vi "Day 10 Task 1 and 2.vi"() -> ()   [LabVIEW 2018]
panel:
  out "Middle score pt2":u64
  out "Scores of incomplete":u64[](array[numeric])
  out "Size of input":i32
  out "Total score pt 1":i64
  out "Scores":i32[](array[numeric])
  out "Error reason":string[](array[string])
  out "Error":bool[](array[boolean])
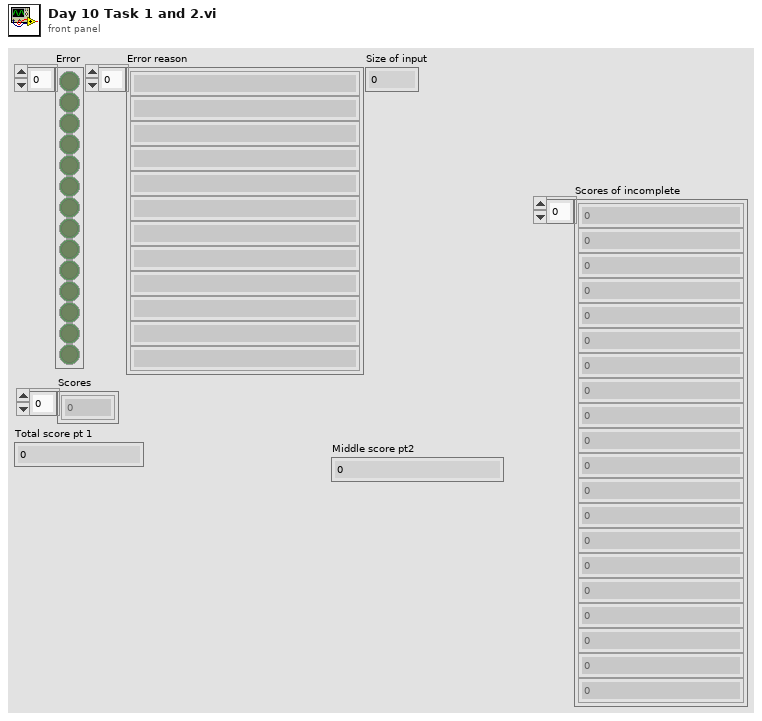
[diagram p1: front panel]
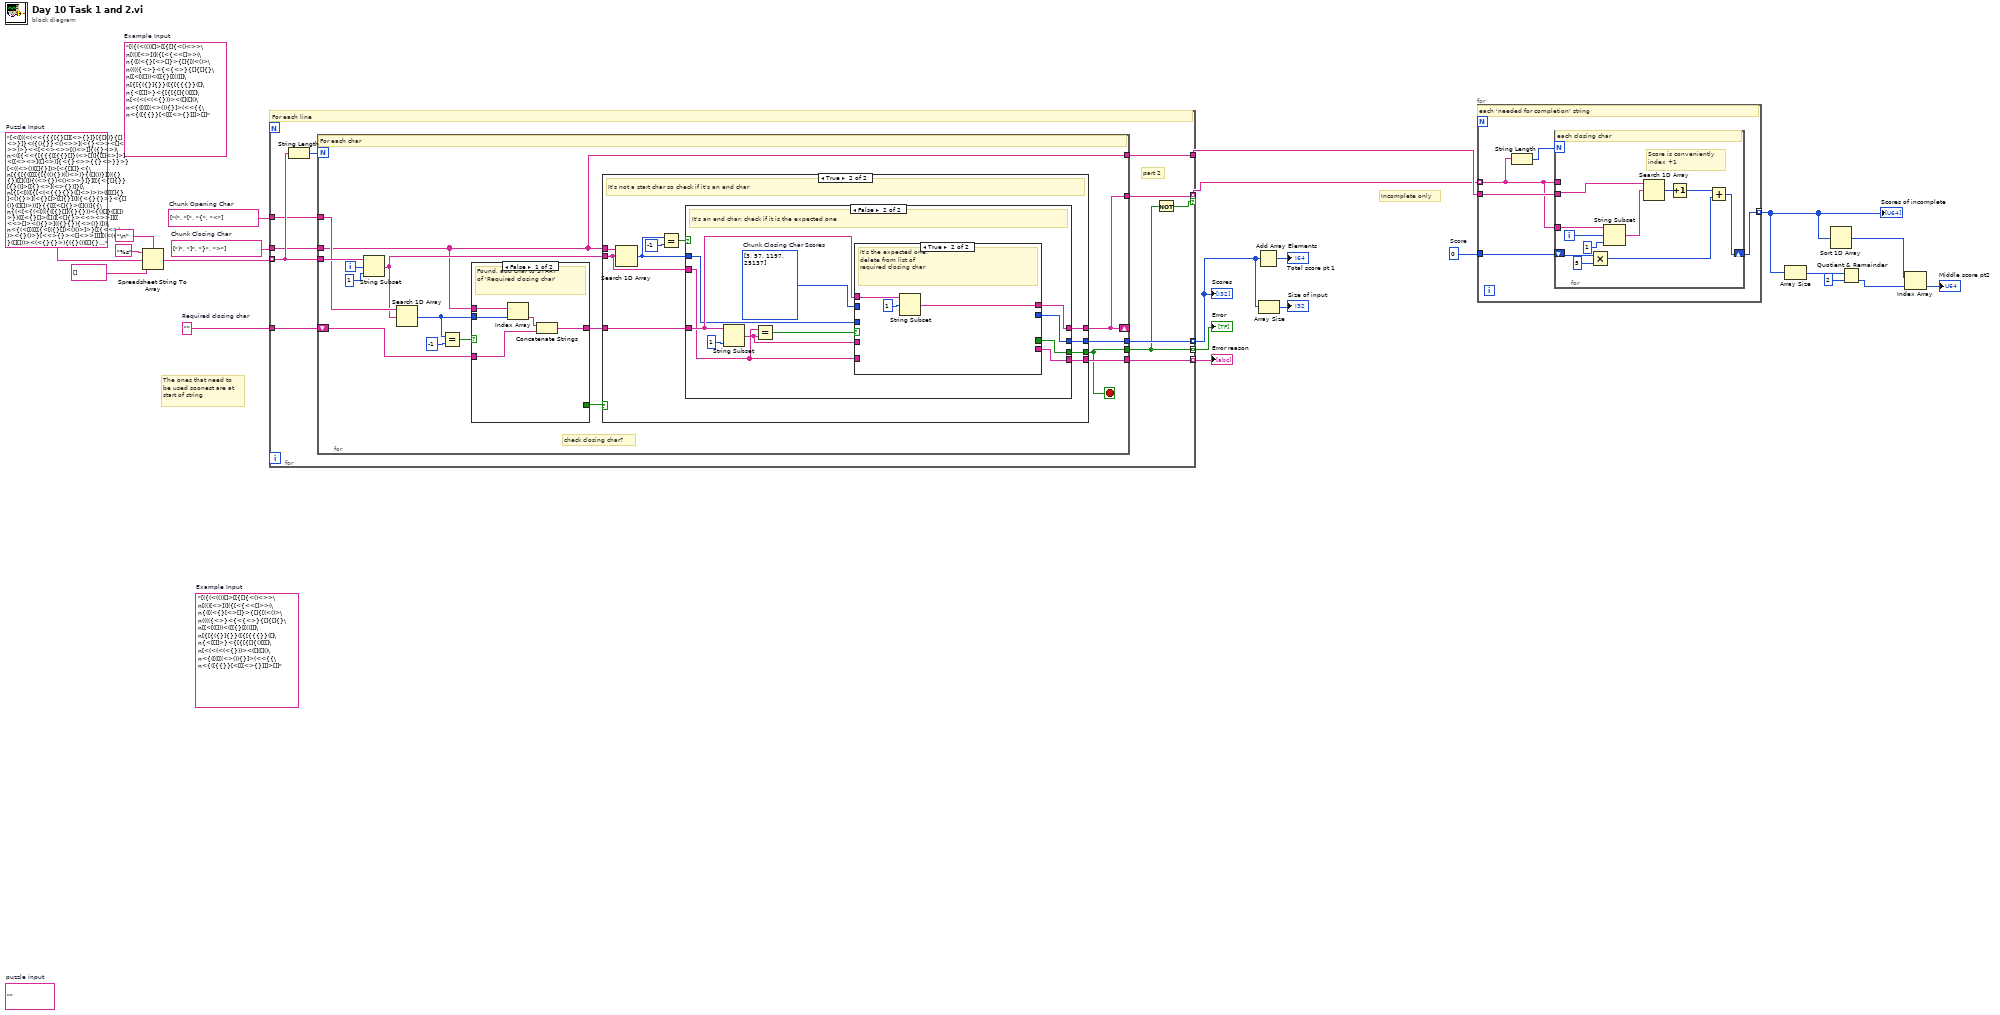
[diagram p0: block diagram]
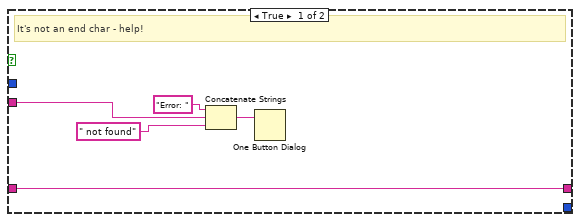
[diagram p3: hidden frame]
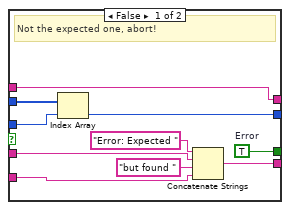
[diagram p4: hidden frame]
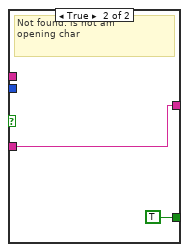
[diagram p5: hidden frame]
diagram:
  w8 = u64 0  # Score
  (unwired) "[({(<(())[]>[[{[]{<()<>>\n[(()[<>])]({[<{<<[]>>(\n{([(<{}[<>[]}>{[]{[(<()>\n(((({<>}<{<{<>}{[]{[]{}\n[[<[([]))<([[{}[[()]]]\n[{[{({}]{}}([{[{{{}}([]\n{<[[]]>}<{[{[{[]{()[[[]\n[<(<(<(<{}))><([]([]()\n<{([([[(<>()){}]>(<<{{\n<{([{{}}[<[[[<>{}]]]>[]]"  # Example Input
  w12 = ""  # Required closing char
  w1 = "[<([((<(<<{{{[{}[]][<>{}]}[{[]()}{[]<>}]}<({(){}}<()<>>](<{}<>><[]<>>)>}<<[<<><>>[()<>]]{({}<>)\n<([{<<{[{{{[[{{}[]}(<>[])]{[[]<>]>]<[[<><>]([]<>)]{<{}<>>{{}<>}}>}[<((<>())[[]{}])>[<{[][]}<{\n[{{[{([[[[{[{((){})(()<>)}{([]())}][(({}{})[[]()]){(<>{})<()<>>}]}][[{<{[]{}}[{}()]>[[{}<>](<>{})]}[\n[{[<[(([{[<(<{{}{}}([]<>)>)>([[[[]{}]<(){}>](<{}[]>[[]{}])]({<{}{}>}<{[]()}([][])>))]}{{[[[<[]{}>([]())]{{\n{(<[<{(<[(({([{}[]]({}{}))<{()[]}([][])>})([[<{}[]>([])][<[]{}><<><>>]][[<<>[]><(){}>](({}{}){<>()})]))\n<{(<[[([[[{<[({}[])<()()>]>}[[{<<>()><{}()>}[<<>{}><[]<>>]]]][(<({[]}([][]))><(<{}{}>){({}())[[]{}]}>){[[\n(<(<(((<<{[<[{[]{}}({}{}>]><[<()<>><{}{}>][{()<>}({}())]>]}({<[[[]()]{[]<>}](<[]<>>([]<>))>[{(<><>)([][])}]\n<{[[{({<([[<{(<>())[<>[]]}><({[]{}}<<>>)[((){})[[]()]]>]]({<<(<><>)[{}<>]>{[{}{}](()[])}>([([]<>){()\n(((<{{{{<<[<([[]<>])({()<>}[{}<>])>(<{<>()}>{[{}<>]})]><[[([[]{}]{{}()})(([]){(){}})]{[{<>{}}<<>{}>\n[{((({[[([[[{{[]<>}(<>[])}[([]{})([][])}]<[(<><>){[][]}]{<{}{}>(()())}>]]<([<{{}()}{{}<>}>[(\n{(<{[[{(<[[{{[(){}](()[])}}<[(<>{}){[][]}]{<<><>>{{}()}}>][{{{()}<()()>}{<<>()>(()[])}}]]>[{<({[<>\n(([([([(([<([([][])<()()>]<({}()]({}())>)>{[{<[][]>(<>{})}<{{}{}}(<>{})>]<{([]())(<>{})}[{<>{}}[()()]]\n{<<<{[({(<({(<{}()>){[<>()](()<>)}})<[<{()[]}{<><>}>]{[[(){}]({}<>)][<<>{}><{}<>>]}>><(([<{}[]>(<>\n{[[([[([{[(<<(<>[]){{}}><([]<>)<()<>>>><([(){}](<>{}))[{[]}<{}<>>]>)][{{(({}())[[]{}])}{([()<>][[]<>]){<[][]>\n{([{(({<<{<{{(<>())[{}{}]}{(()[])[[]<>]}}>}>[<{(<[[]()]<{}()>>)<{((){}]((){})}[[{}]([]{})]>}([({\n(([(<({[<({{<{<>[]}<<>{}>](([]()))}<(<{}()>(<>))<((){})[<>{}]>>})({[[<()<>>][<()<>>[<><>]]](({\n<<((<<{[{(<<<{{}{}}[{}<>])(<<>()>[[][]])>>([({()[]}[<>{}]){[{}<>]{()<>}}]{(<{}{}>[<>[]])[{<>[]}<[]{\n([{(<<{{<{<<<<()<>>([][])>(([]()){()})><{[{}()]{<>{}}}<{()<>}<()[]]>>>}{<<<{()}((){})>[[{}()][<>]]>>[\n<[(<<<([{{{((<()>(<>{}))<([]<>)(<>())>){([(){}]<()()>)}}{{[[()[]](()<>)]{(<>()){()()}}}<[({}()){[]<>}][<{}[\n(<{{({({({[{([()<>])[{<>{}}]}{<([]())[[]<>]>([()()]{[]<>})}]{(<[{}()]<<>()>>[<<>())<()[]>])[({()()}[[]\n<({<({[{(({{{<{}()>[(){}]}{({}<>)<[]{}>}}<<<{}[]>([]<>)>[(()())[()<>]]>}<(<[[]{}]([]())>([(){}]<[][]\n{(((<(<{{{<[[{[][]}]<{[]{})[{}()]>]<[<{}<>>][[[]()](()<>)]>>}([([{{}[]}[<>[]]][(<>{}){[]()}])({[{}[]][<>\n{{({(<{{(([<(<()<>>{(){}})>[<{()()}[<>{}]>[<<>{}>{[][]}]]]({{<<><>><[][]>}[[<>()]<[]()>>}<<(()())[[]<>]><{<\n<{(<([{[{<[[[(<>)({}{})]]((<()<>>))]{{{(()<>)([])}}[{{{}()}{<>[]}}[{[]{}}{<><>}]]}>}][<[<[<[(){}]><({}[])<<>{\n<({[[<<([(<{[<[]<>>[{}<>]](({}[]))}{{[{}<>]}([[]{}]([]{}))}>[[{<[]<>)<{}>}{{(){}}{()}}]([(<>{})]<<[]()>\n{(([{<{(((<<<(()[])([]())>[<<>{}>({}[]]]>>[[([[]<>]<{}[]>)<[<>[]]{(){}}>][((<>[])(()[]))]]))(([{<{<>}{{}<>\n<[((([<{{([{({<>{}}(<><>)){([]{})<()[]>}}({[[][]]([]{})}({[]<>}))][<<[<>{}]([][])>(<{}<>>[(\n<[{{[{{<{[[([<<><>>]{({}())([]<>)})]]}[<({([{}{}]{[]})({()()}[(){}])}[{<(){}><{}[]>}])<[[<[]{}>\n(<(<{<{<{([([<<><>>]({[]}[()[]])){<{<>()}<()[]>>[([]{}){{}[]}]}]{{({[]()}{<><>})([{}()](()()))}<[<[][]>][<[]\n{[{{<[(<(<{<{{<><>}{{}{}}}([()()])>[<<{}>[()()]>[[()()]{[][]}]]}>)[<<<<<[]()><(){}>>[[<>()]<{}{}>]>[{{\n([{(<({((([<(<()()><[]()>)({{}()}{<>()})>{[({}[]){{}[]}]{{{}()}{{}<>}}}])(<[{((){}){[][]}}([[]()])]{<{()<>\n((<<[{<[(([({(()<>)[{}{}]}{<{}[]><[]<>>})<[<()>]([()<>])>]{((<[]{}><()<>>)<{{}><<>>>)[(<{}()>)<[[]()](\n({<([[<{[{[[{{{}<>}({}())}<[<>()][{}[]]]][[{[]<>}]<([]{})[{}()]>]]}]([{[(<[]{}>[{}[]])]}]{((<[{}\n<[(<{<[<<({<<{<><>}(()())>)}{(({(){}}){[{}[]]{{}{}}})})>>]>}<[<{(<<[(<()<>>[[]()]){{{}<>}<[][]>}][(<(\n({([(<{[{[{<({<>{}}<()[]>)>{[(<><>){{}<>}]}}]}]}[([[{[[[[]{}]][([][]){<>{}}]][[{[][]}(<>[])]\n[<([<[([[{{({{<>{}}[{}[]]}([()()]({})))((<(){}>)([[]())({}<>)))}}]])]>{<<(({{<[<{}[]>[()<>]]>}}([[{({}<>)\n<{[{<[<([{(<{<<>{}><<>()>}[(<>[])[<><>]]>[(((){}))<(<>){{}[]}>]){(<({}{})[{}{}]}<<[]{}><{}<>>>\n{[[{<{[<<<(<<(<><>)<[][]>>{[<>{}]{()<>}}>{{{[]<>}<<>()>}}){(<{<>()}(()<>)>{{{}[]}(()())})]>>({(([<{}()>([]{\n[<({(({<<{<<{<<>>{<><>}}((<>{})({}()))>([({}())([][])][{{}{}}<[]<>>])>}((<<<(){}>{{}()}>[{<>()}({}{\n<([[[{[(({([{<()<>>}]{(([]<>)[()<>])}){<[{()()}[<><>]]([<><>][{}[]])>{({{}{}}){<{}[]><<><>>}}}}{<({<()<>\n<[<((<[[<({{[{<><>}{{}{}}]{<{}{}><(){}>}}{{[[]{}][<>[]]}([<><>][{}()])}}({{{<>()}<<>{}>}([{}]{\n{[(<({[{<<{<{{()[]}({}())}{{{}()}<()>}>[<([]{})<<>{}>><{{}()}{{}{}}>]}<{({[][]}{{}[]})}<<{<>{}}[[][]]>>>>\n<{[<([(<<([[(<[]<>><{}()>)<({}<>){(){}}>]]<<[(<>{}){{}<>}]([[]{}]({}{}))>>)>{[{[<<[]><{}<>>>(({}{}))\n{(<<{{{((<<[({[][]})[([]())(<>{})]][((()<>)([][]))}><([[()[]]]){<<[][]>><<{}[]>[(){}]>}>>[([{[[]<\n<{(<<<{{((<{{<{}()>[<>()]}({<>{}}[(){}])}[{({}<>)(()[])}<{(){}}<{}{}>>]>{{[[[]{}]<[][]>]{[{}{}][[]<>]}\n{(<(<([{<([<{{<>}<<>{}>}{<()[]>[[]()]}>{<[()()]({}{})>((<>{}))}][{<{[]}[[]()]>{{<>}[[]<>]}}({<<>{}>[[][]]}{<\n{((<[<<[{<{[{{{}<>}}<[<>()]([]())>]([<()()><()()>]{[()<>]{[]()}})}<{([[]()]{<>})}(<<[]{}}{[][\n[{{{<<<[{[(<[{[]{}}{(){}}}(<()>[[][]])>{{(<><>)<<>()>}<<<>{}>(())>})]{<(<<[]()>({}())><[{}<>]{[]()}>)><\n{{[[[({((({{({{}()}<()()>)}{(<{}{}>{()<>})[(()<>)<<><>>]}}<[<[{}[]][()<>]>[[(){}][()()]]>{<{<>[]}[\n[<[([{[{[{[{({(){}})}[[<[]{}>{<>()}]]]<[<{<>()}[<><>]>[{<>[]}<()()>]][<{[]{}}({}())>{<[]()>{{}()}}]>\n<([{({<(({<{<[[]{}]({}[])>[[<>[]]<<>[]>]}>}{(({(()[])[[]()]})<[[{}<>][<>{}]]<[[]()]([])>>)}))[([[([([][])[<\n{<{[([(({<(<{{<>[]}[[]<>]}<(<><>)[[]{}]>>{{{{}()}((){})}))<[{[{}{}]([]{})}{([]())(<>{})}][<(()[])\n([[[([<[[{{((<{}{}>(<>()))[({}[]){<>{}}])}}[[(({{}{}}(()[]))<[<>{}]<()<>>>)]<({<()<>>}{{{}<>}{(\n(<([{[{<[{[<<<{}()}{{}<>}>({(){}}<[][]>)><{<<>[]>((){})}>](<([()()])[([])({}{})]>[[<{}[]>(<>\n([(<{<([{{[[[({}{})[(){}]]]([(()<>)[<>[]]][<{}{}>])][<[<<>[]>[(){}]][[{}[]](<>[])]>({{{}[]>([]{})}[{[][]}[{}\n{<[(<[({[<({[({}[])]<{{}<>}[{}()]>}<{{{}{}}[[]]}<(()())[[]<>]>>)>{[{[(<>{})[<>{}]]<({}<>)((){})\n{[{[<<<[([[[<{[]{}}[<>()]>(([][])({}[]))]<[[<>()]{<>()}]<[()[]]{[]()}>>]](<{<[()[]]>{({}{})}}(<<[]<>><[]<>>\n({[<{{<<({<(<[{}{}]>)[(<{}{}>[[]{}]){<{}()>{<>[]}}]>(({<<><>><<><>>}({[][]}))[[{{}}([]{})]])}[({(<{}[]>{()<>}\n({{{{{{[<[<([([]){{}[]}][([]{})])(<([]{})(<>{})><[<>](()())>)>{(([[]()](()())))}]{[[({()[]}{<>(\n(({{[<[[[((<{(()<>)[[]{}]}([[]()]{<><>})>))((<{{(){}}(<>())}(<<><>><[]{}>)>(({()()}[{}[]])))<([<<>><()[]>])<\n<[[{<({[((<<({{}()}{<><>})<<()[]>[{}()]>>><(<[[][]][()]><[()[]]>)>>){{<((({}<>)(()))(<{}()>)\n{<{[([{<{<([{[<>{}][{}{}]}[([]())[[]<>]]]{([<><>]<<>{}})}){[(([][]){<><>}){<<>{}>[()[]]}]<(<()()>{{}})<([]\n<{<{<([[[[{[({[][]}<[]{}>){[<>{}]{[]}}]}([[(<>[])][(<><>)<<>{}>]]<([()<>][()()])[<[]()><<>\n(<((({{{<([{<[()()]{[]()}>[{{}{}}[()[]]]}]{[(<()<>><[]{}>)<<{}()>[<>[]]}]([[()()]]{(()<>)})}){<{{({}())(\n[[[[(([{[(((((<>()){{}{}})(<[]()>({}<>)))<<<()>([]>>((()<>)[<><>])>)([[<()[]><{}()>]{{[][]}([]<\n[[{([(<((<[[(([]<>)({}[]))<(())>]]>))>(<([[<{((){})<<>{}>}>{{<()()>[<>[]]}([[]{}]{[][]})}]])[<[<\n((([[(<(<[<((<{}()>({}[]))<<<>[]>[()[]]>)([((){})({}())])>][<[(<()()>{{}{}}){<{}<>>{()[]}}]>{[{{{}(\n{<(([((<[({<<{<>[]}[[]()]>>([<{}{}]({}())]([()()]<{}<>>))}({[<()()>{[]{}}]((()<>)<()()>)}))([<[[<><>\n<[{[<{({([{([({}<>)({}{}>])<([{}{}][()[]])<([]())>>}[{<(<>{})((){})><[<><>](()[])>}<<{<>{}}([])><({}(\n({{<<<(([<{<<([]<>)[<>]][{[]{}}{(){}}]>{(({}{}){()<>})}}[({<{}()><(){}>}{([]{})[<>[]]})<[{<>\n(<<(<[({[<({<<()<>>({}<>)>})<({<()()><{}{}>}[{(){}}[<><>]]){(({}())<{}<>>)<<(){}>({}<>)>}>>((((<<\n[{{{({[{([<<<(<><>)<{}<>>>{{[]()}[()[]]}>{[<<>{}><<>[]>]{[[]{}][()<>]}}>{<<[()<>]><([]{}){<><>}>>[{{{}()}{()[\n[[{{(<[[{<<[<[{}{}][{}{}]>>({[(){}]<{}{}>}(((){})[<>[]]))>>}((({<(()<>){{}{}}>{<()[]>[{}[]]}}\n(((<{{<{[<<[{{[][]}{[][]}}]{[{[]<>}{()}]}>{{[[[]<>]<(){}>]<[[]()][[]()]>}[<<[]<>>(<>}>{(()<>)<()()>}]}>[\n([[{[({{{{[(<<()<>>(<>[])>[(()())<[]{}>])]<{{(<><>)(()<>)}([<><>]<(){}>>}>}[<{({(){}}<()<>>){(<><\n{({<{[(<{(({<[[]{}](()())>(((){}))})<(<{<>()}<{}>>{<()()>([]{})})([[<>[]]{[]()}][{<>[]}[{}[]]])>)<{<(<{}()>\n{(({[{<{<({{(<[]{}><{}()>)[{{}<>}]}})(<{([()()]{()<>})<{<>()}<[]()>>}<([()[]]([]{}))<{{}{}}<<>[])>>>{({[[]{\n<<{{([([[[{<{[<>()]]>{<[[]{}]((){})>{{<>{}}<{}<>>}}}{{{<<>{}>({}<>)}[<(){}><{}()>]}([<{}<>>(<>[])\n[{<[<{{{{<({{<{}()>{{}<>}}})[(<{<>[]}{<>()}>[(<>())<()>])<<{()[]}<<>()>>{([]<>>}>]><({[[{}[]]\n[{{<(<({(<{[<[<>[]]{()<>}><(<>[]){{}}>]{<<<>{}>[<>{}]><[[]<>]{<>()})}}>)}[[({{<[()()][(){}]>((()[])(\n[[[[[[[[<<([<[()[]](<><>)><(<>[])<<>{}>>])><{[<<<>{}><{}()>>({[][]}<[]{}>)]([{<>()}{{}[]}]{{{}{}}{[]()}}\n<(((<(([<{(<[[[][]]{()[]}]<(<>{}){[]{}}>>)}>]))[({[<<{(<()[]>([]<>))[<()[]>{()[]}]}<([<><>](<>[]))((<>()\n<{{{<{{{[[{([({}{})<[][]>]<[<>{}]{<>()}>)}<({{[]<>}([]())}<<<>[]><<>{}>>){(<[]><(){}>)>>]{{(<([]<>)([](\n<[<{[<{{([(({(<>())}{[<>[]](()<>)})([([][]){<>()}][<[]<>>{[]{}}]))])}([{{(<{<>()}[()<>])((\n{{[({[[{([<<{<()()>[()[]]}{<<>{}>{{}()}}>>]<{<[<{}()>{[][]}][{[][]}[<><>>]>}>)}]][<((({({([]{})\n[(<[([<{[[{{<{{}[]}({}())>([{}[]]{[]})}([([]())<<><>>]<(())<<>>>)}[<[(<>{}){{}<>}]{{()<>}[<>{\n{{[{[<([{<[((<(){}><()[]>){[{}]({}<>)})(([()[]]<<>[]>)<[(){}]>]]{({[<>()][<>[]]}({[]{}}{{}[]}))[[[(){}][[]{}\n{[<<<[<[{[<((<[]{}>)<([]<>){{}<>}>)<{([]())({}{})}>>](<([(<><>)[[]<>]]<{<><>}{()[]}>)>[(<<<>()><()[]>>\n<[<((<<(<{(({<{}<>>{{}<>}}{<[]()>{<>{}}})){<[(<><>)<()<>>]>[{{<>{}}<(){}>}<{<><>}({}())>]}}>)>[[{<[[\n[([((<<([<{<[[()()]][[{}[]]]>{{(<>{})<<>()>][{[]()}]}}>])<([{<({{}()}<<>{}>)><[[()]<()[]>][[()<>](<>\n{{((<[(({<[<[<[]<>>[(){}]](<[]<>><{}[]>)>][({{[]()}{<>[]}}{(()[]){<><>}})<[<{}[]>]>]>}<{[{{{<>[]}{{}()}}{{<>\n({{({{{{{{[<[({}())[<><>]]>[(<<>[]>((){}))]]{{(<<>()>[{}[]])[{<>{}}<{}[]>]}{({{}()})}}}[[({{{}<>}<()()>}({()\n[<<[((({<<<(({(){}}({}{})){<<>{}>{{}{}}}]((<[][]>{<>[]}))>>{[[([()()])<[()[]]{[]<>}>][(<<>()>({}[]))<({}[]\n{(<<(<{({<<[[(<><>){(){}}][([]())([][])]](<<<>()>[[][]]>[({}{})[()<>]])>((<[[]<>]<{}()>>){<([][])[[]<>\n<([{<[({{{[<{{()<>}(<><>)}{<{}()>[{}<>]}>{{[{}{}]<<>>}<[<>()]<<>[]>>}]{<<([][]){[]()}>[<{}()><()()>]>[\n(<<[[<(<{[<(([()<>]<()<>>){[{}[]][{}()]})<[[<><>]<[]>]<[[]()]{[]{}}>>>}<[[[<{}{}>(<>())]]{({<>{}}([\n[(([<(<(([(<<<{}{}>[[]()]>[<[][]>{[]}]><<<<>()>[[]{}]>([[][]]{<>()})>)(({<<><>>[()()]}))]))>((({((\n<<[[<{{({[{({(<><>)(()<>)}[[<><>]])[({<><>}([][]))[[[]()]([]{})]]}]<{({(<>{})[(){}]}({()<>}))([{(\n({[<<<<[<(<[<[[]<>]([]<>)>{<(){}><[]()>}]{[(()<>)(()())][{(){}}[<>]]}>)>][(([({([][])<[][]>][{(){}}({})])<<{[\n<<({[(<{<(<({<[]<>>{()()}})<{<()[]>[[]()]}(((){}){<>})>>){[[<[{}()]>][{[(){}]({}[])}<[<>[]](<><>)>]]({(<<\n<[([[(<<({(<<({}())]>{[[[]<>][[]()]]})<<{([]())[[]<>]}<(())<{}<>>>>{(([]{}){<>{}}){[{}()][(){}]}}>})><\n{(<{{[{<({[[[[{}()]({}[])]({()()}{{}[]})]{<[(){}]>([{}()]{{}{}})}](<{<{}[]>[{}[]]}((()[]){<>{}})>([{[]{\n<[(<({<(<[<{<([]<>)<<><>>>([<><>])}>]{([{(<><>)(<>())}[{()()}{(){}}]]){{{([]{}}{{}[]}}<{<>[]}[[\n<[<[[{([<({([<[]()><[]<>>])[([[]<>]{{}})]}<<<<[]<>>(()[])>({()()}<<>[]>)>[<{[]<>}>({()()}(()<>))]>)({(\n{{<[(<{{{<[<(([]<>}[<>{}])><<<<>{}>([]())>[([][])]>]>}}}>)]>(({(<{<<<(({()}<[][]>)[<[]>{<><>}\n({{[<[({[[{({{{}[])}<[<>[]][<><>]>)<{{[]{}}{{}[]}}>}]<((<(<>()){()}>)(<[{}()]{<><>}>(<()()>{()[]})"  # Puzzle Input
  w18 = string[] [")", "]", "}", ">"]  # Chunk Closing Char
  w11 = string[] ["(", "[", "{", "<"]  # Chunk Opening Char
  (unwired) ""  # puzzle input
  (unwired) "[({(<(())[]>[[{[]{<()<>>\n[(()[<>])]({[<{<<[]>>(\n{([(<{}[<>[]}>{[]{[(<()>\n(((({<>}<{<{<>}{[]{[]{}\n[[<[([]))<([[{}[[()]]]\n[{[{({}]{}}([{[{{{}}([]\n{<[[]]>}<{[{[{[]{()[[[]\n[<(<(<(<{}))><([]([]()\n<{([([[(<>()){}]>(<<{{\n<{([{{}}[<[[[<>{}]]]>[]]"  # Example Input
  # "Incomplete only"
  # "The ones that need to \nbe used soonest are at\nstart of string"
  n1 = Spreadsheet String To Array(delimiter (Tab)="\n", format string="%s", spreadsheet string=w1, array type (2D Dbl)=string[] []) -> (array=w19:string[])
  n2 = for {
    tunnel: w19 -> [w29] mode=indexing
    tunnel: w11 -> [w28]
    tunnel: w18 -> [w27]
    tunnel: [w25] -> w17 mode=indexing
    tunnel: [w32] -> w16 mode=indexing
    tunnel: [w31] -> w14 mode=indexing
    tunnel: w12 -> [w30]
    tunnel: [w24] -> w9 mode=indexing if=w26
    tunnel: [w23] -> w10
    # "part 2"
    # "For each line"
    n3 = String Length(string=w29) -> (length=w33:i32)
    n4 = for {
      N: w33 -> [_]
      tunnel: w29 -> [w49]
      tunnel: w27 -> [w34]
      tunnel: w28 -> [w46]
      shift-right: [w36] -> _
      shift-left: w30 -> [w45]
      tunnel: [w35] -> w25
      tunnel: [w38] -> w32
      tunnel: [w37] -> w31
      tunnel: [w36] -> w24
      tunnel: [w34] -> w23
      i -> [w48]
      stop <- w35 stop-if-true
      # "check closing char?"
      # "For each char"
      n5 = String Subset(string=w49, offset (0)=w48, length (rest)=1 ("length (rest)")) -> (substring=w41:string)
      n6 = Search 1D Array(1D array=w46, element=w41) -> (index of element=w39:i32)  [unwired: 1 in]
      n7 = Equal?(x=w39, y=-1) -> (x = y?=w43:bool)
      n8 = case shown="False" w43 {
        tunnel: w34 -> [w94 _]
        tunnel: w45 -> [w92 w96]
        tunnel: [w91 w96] -> w40
        tunnel: [_ TRUE ("Check closing char")] -> w42
        tunnel: w39 -> [w90 _]
        frame False {
          # "Found, add char to START\nof 'Required closing char'"
          n9 = Index Array(array=w94, index=w90) -> (element=w93:string)
          n10 = Concatenate Strings(w93, w92) -> (w91:string)
        }
        frame True {
          # "Not found: is not am\nopening char"
        }
      }
      n11 = case shown="True" w42 {
        tunnel: w34 -> [_ w60]
        tunnel: w41 -> [_ w57]
        tunnel: w40 -> [w50 w56]
        tunnel: [_ w55] -> w35
        tunnel: [w50 w54] -> w36
        tunnel: [_ w53] -> w38
        tunnel: [_ w51] -> w37
        frame False {
          # "It was a start char so no need to search end char"
        }
        frame True {
          # "It's not a start char so check if it's an end char"
          n12 = Search 1D Array(1D array=w60, element=w57) -> (index of element=w52:i32)  [unwired: 1 in]
          n13 = Equal?(x=w52, y=-1) -> (x = y?=w58:bool)
          n14 = case shown="False" w58 {
            tunnel: w57 -> [w65 w71]
            tunnel: w56 -> [w61 w73]
            tunnel: [_ w74] -> w55
            tunnel: [w61 w72] -> w54
            tunnel: [_ w69] -> w53
            tunnel: w52 -> [_ w68]
            tunnel: [_ w66] -> w51
            frame True {
              # "It's not an end char - help!"
              n15 = Concatenate Strings("Error: " ("string"), w65, " not found" ("string")) -> (w64:string)
              n16 = One Button Dialog(message=w64) -> ()  [unwired: 1 in, 1 out]
            }
            frame False {
              w67 = i32[] [3, 57, 1197, 25137]  # Chunk Closing Char Scores
              # "It's an end char: check if it is the expected one"
              n17 = String Subset(string=w73, length (rest)=1 ("length (rest)")) -> (substring=w70:string)  [unwired: 1 in]
              n18 = Equal?(x=w71, y=w70) -> (x = y?=w75:bool)
              n19 = case shown="True" w75 {
                tunnel: [w86 _] -> w74
                tunnel: w73 -> [w83 w88]
                tunnel: [w83 w87] -> w72
                tunnel: w71 -> [w82 _]
                tunnel: w70 -> [w81 _]
                tunnel: [w80 _] -> w69
                tunnel: w68 -> [w79 _]
                tunnel: w67 -> [w78 _]
                tunnel: [w77 _] -> w66
                frame False {
                  w86 = TRUE  # Error
                  # "Not the expected one, abort!"
                  n20 = Index Array(array=w78, index=w79) -> (element=w77:i32)
                  n21 = Concatenate Strings("Error: Expected " ("string"), w81, "but found " ("string"), w82) -> (w80:string)
                }
                frame True {
                  # "It's the expected one, \ndelete from list of\nrequired closing char"
                  n22 = String Subset(string=w88, offset (0)=1) -> (substring=w87:string)  [unwired: 1 in]
                }
              }
            }
          }
        }
      }
    }
    n23 = Not(x=w25) -> (.not. x?=w26:bool)
  }
  "Error" <- w17
  "Error reason" <- w16
  "Scores" <- w14
  n24 = Add Array Elements(numeric array=w14) -> (sum=→"Total score pt 1":i32)
  n25 = Array Size(array=w14) -> (size(s)=→"Size of input":i32)
  n26 = for {
    tunnel: w10 -> [w101]
    tunnel: w9 -> [w99] mode=indexing
    tunnel: w8 -> [w97]
    tunnel: [w100] -> w4 mode=indexing
    # "each 'needed for completion' string"
    n27 = String Length(string=w99) -> (length=w98:i32)
    n28 = for {
      N: w98 -> [_]
      tunnel: w101 -> [w112]
      tunnel: w99 -> [_]
      tunnel: w99 -> [w110]
      shift-right: [w105] -> w100
      shift-left: w97 -> [w104]
      i -> [w109]
      # "Score is conveniently\nindex +1"
      # "each closing char"
      n29 = Multiply(x=w104, y=u64 5) -> (x*y=w102:u64)
      n30 = String Subset(string=w110, offset (0)=w109, length (rest)=1 ("length (rest)")) -> (substring=w107:string)
      n31 = Search 1D Array(1D array=w112, element=w107) -> (index of element=w111:i32)  [unwired: 1 in]
      n32 = Increment(x=w111) -> (x+1=w106:i32)
      n33 = Add(x=w106, y=w102) -> (x+y=w105:u64)
    }
  }
  "Scores of incomplete" <- w4
  n34 = Array Size(array=w4) -> (size(s)=w7:i32)
  n35 = Sort 1D Array(array=w4) -> (sorted array=w3:u64[])
  n36 = Quotient & Remainder(x=w7, y=2) -> (floor(x/y)=w5:i32)  [unwired: 1 out]
  n37 = Index Array(array=w3, index=w5) -> (element=→"Middle score pt2":u64)
